vi "TSLIN_Funtion_test.vi"() -> ()   [LabVIEW 2014]
uses:
  Utilities/Typedef/Hardware_Subtype.ctl
panel:
  in  "Hardware Subtype":T1=enum."TC1016"
  in  "AHwCh":i32(ring) items=["CHN1", "CHN2", "CHN3", "CHN4", "CHN5", "CHN6", "CHN7", "CHN8", "CHN9", "CHN10", "CHN11", "CHN12", "CHN13", "CHN14", "CHN15", "CHN16", "CHN17", "CHN18", "CHN19", "CHN20", "CHN21", "CHN22", "CHN23", "CHN24", "CHN25", "CHN26", "CHN27", "CHN28", "CHN29", "CHN30", "CHN31", "CHN32"]
  in  "AAppCh":i32(ring) items=["CHN1", "CHN2", "CHN3", "CHN4", "CHN5", "CHN6", "CHN7", "CHN8", "CHN9", "CHN10", "CHN11", "CHN12", "CHN13", "CHN14", "CHN15", "CHN16", "CHN17", "CHN18", "CHN19", "CHN20", "CHN21", "CHN22", "CHN23", "CHN24", "CHN25", "CHN26", "CHN27", "CHN28", "CHN29", "CHN30", "CHN31", "CHN32"]
  in  "Baudrate":sgl=19.2 format="%#_g  k"
  in  "Protocol":i32(ring)=2 items=["Lin_Protocol_13", "Lin_Protocol_20", "Lin_Protocol_21", "Lin_Protocol_J2602"]
  in  "Channels used":u16(ring)=1 items=["1 Channel"=1, "2 Channels"=2, "3 Channels"=3, "4 Channels"=4, "5 Channels"=5, "6 Channels"=6, "7 Channels"=7, "8 Channels"=8, "9 Channels"=9, "10 Channels"=10, "11 Channels"=11, "12 Channels"=12, "13 Channels"=13, "14 Channels"=14, "15 Channels"=15]
  out "Connect ?":bool
  in  "Disconnect":bool
  in  "Connect":bool
  in  "Config":bool
  in  "DLL_PATH":path
  in  "停止按钮":bool
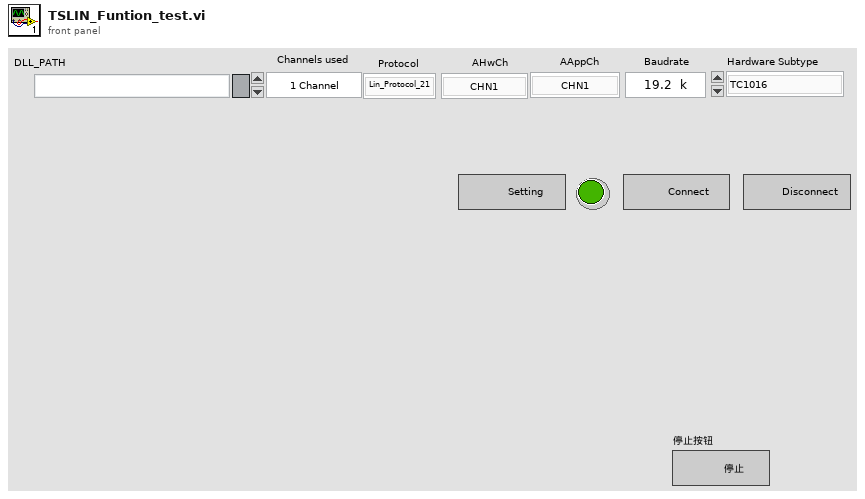
[diagram p1: front panel]
types:
  T1 = typedef "Hardware_Subtype.ctl" = enum16{"TS_UNKNOWN_DEVICE", "TSCAN_PRO", "TSCAN_Lite1", "TC1001", "TL1001", "TC1011", "TM5011", "TC1002", "TC1014", "TSCANFD2517", "TC1026", "TC1016", "TC1012", "TC1013", "TLog1002", "TC1034", "TC1018", "GW2116", "TC2115", "MP1013", "TC1113", "TC1114", "TP1013", "TC1017", "TP1018", "TF10XX", "TL1004_FD_4_LIN_2", "TE1051", "TP1051", "TP1034", "TTS9015", "TP1026", "TTS1026", "TTS1034", "TTS1018", "TL1011", "TTS1015_LiAuto", "TTS1013_LiAuto", "TTS1016Pro", "TC1054Pro", "TC1054", "TLog1038", "TO1013", "TC1034Pro", "TC1018Pro", "TC1038Pro", "TS_DEV_END"}
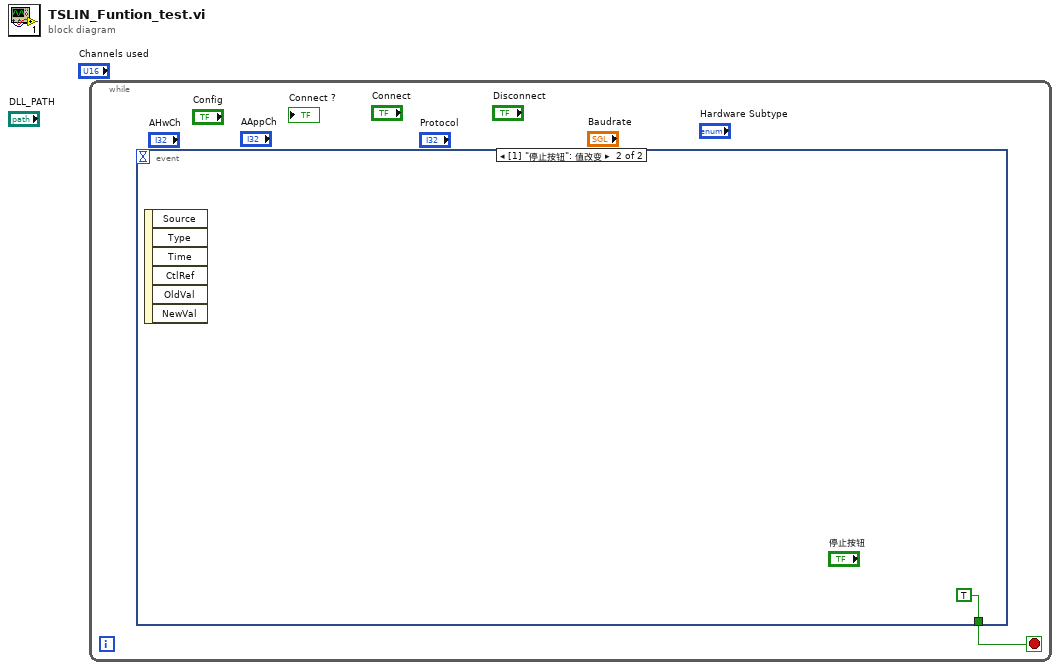
[diagram p0: block diagram]
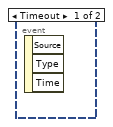
[diagram p2: hidden frame]
diagram:
  n1 = while {
    stop <- w1 stop-if-true
    n2 = event shown="[1] \"停止按钮\": 值改变" {
      selector: _ -> [_ _]
      dyn-events: _ -> [_ _]
      timeout: _ -> [_ _]
      tunnel: [_ TRUE] -> w1
      event Timeout {
        n3 = event-data() -> ()  [unwired: 1 in, 3 out]
      }
      event "停止按钮": Value Change {
        n4 = event-data() -> ()  [unwired: 1 in, 6 out]
      }
    }
  }
